vi "Regular Expression Test.vi"() -> ()   [LabVIEW 2015]
uses:
  <vilib>/regexp/Match Regular Expression.xnode
panel:
  out "submatch 3":string
  out "submatch 2":string
  out "error out":errorcluster
  out "submatch 1":string
  out "after match":string
  out "whole match":string
  out "before match":string
  in  "string":string
  in  "regular expression":string="[\\d\\w]+]/port[\\d]"
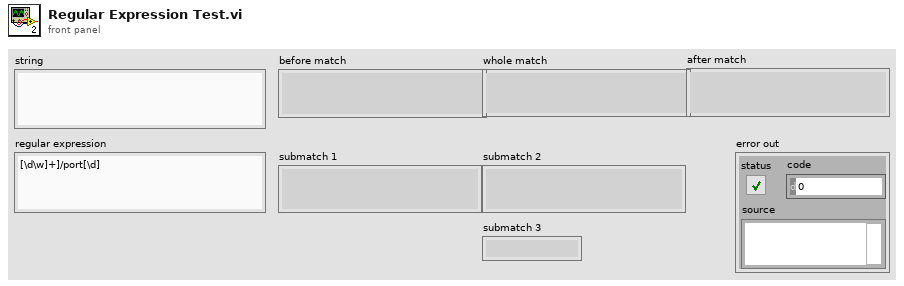
[diagram p1: front panel]
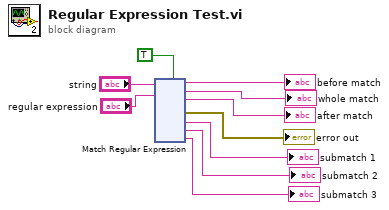
[diagram p0: block diagram]
diagram:
  n1 = xnode "Match Regular Expression"("input string"="string", "regular expression"="regular expression", "multiline? (F)"=TRUE) -> ("before match"=→"before match":string, "whole match"=→"whole match":string, "after match"=→"after match":string, "error out"=→"error out":errorcluster, "submatch 1"=→"submatch 1":string, "submatch 2"=→"submatch 2":string, "submatch 3"=→"submatch 3":string)  [unwired: 3 in, 1 out]
